vi "Byte Buffer.Read (1D I8).vi"(7 "byte order (big-endian)":T1(ring), 8 "error in (no error)":errorcluster, 9 "count":i32, 10 "buffer offset":i32, 11 "buffer in":string) -> (0 "error out":errorcluster, 1 "value":i8[](array[numeric]), 3 "buffer out":string)   [LabVIEW 2016, in "VeriStand Data.lvlib"]
doc: "Reads <B>count</B> elements of data from the provided <B>buffer</B> at location <B>buffer offset</B> in the format of the data type specified. The data endianness can be specified via <B>byte order</B>."
uses:
  VeriStand Data.lvlib
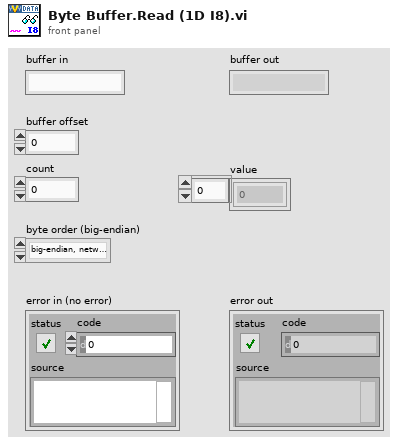
[diagram p1: front panel]
types:
  T1 = enum16{"big-endian, network order", "native, host order", "little-endian"}
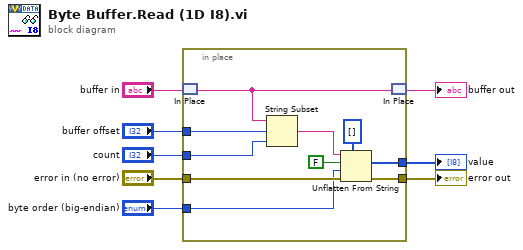
[diagram p0: block diagram]
diagram:
  n1 = in-place {
    in-place-border: "buffer offset" -> [w17]
    in-place-border: "error in (no error)" -> [w15]
    in-place-border: "byte order (big-endian)" -> [w13]
    in-place-border: [w11] -> w4
    in-place-border: [w10] -> w2
    in-place-border: "count" -> [w9]
    n2 = in-place-match #1("buffer in") -> (w18:string)
    n3 = String Subset(string=w18, offset (0)=w17, length (rest)=w9) -> (substring=w16:string)
    n4 = Unflatten From String(type=i8[] [], binary string=w16, data includes array or string size? (T)=FALSE, byte order (0:big-endian, network order)=w13, error in (no error)=w15) -> (value=w10:i8[], error out=w11:errorcluster)  [unwired: 1 out]
    n5 = in-place-match #1(w18) -> (→"buffer out":string)
  }
  "value" <- w2
  "error out" <- w4
